vi "GA_Insert Into Population.vi"(6 "Parameters":T3={"Population size"=100, "Generations no."=500, "Significant digits"=4, "Crossover probabality"=0.85, "Mutation mode"=enum."one-point, fixed rate", "Use Gray code?"=FALSE, "Mutation rate"=0.05, "Min mutation rate"=0.0005, "Max mutation rate"=0.25, "Reproduction plan"=enum."Steady-state-replace-worst", "Elitism"=FALSE, "Fmax"=1} {"Max mutation rate" min=0.0 max=1.0; "Min mutation rate" min=0.0 max=1.0; "Mutation rate" min=0.0 max=1.0; "Crossover probabality" min=0.0 max=1.0; "Significant digits" min=1; "Generations no." min=1; "Population size" min=1}, 7 "Fitness Function":T2, 8 "Offsprings":i32[][](array[numeric]), 11 "Population in":T1) -> (3 "Population out":T1)   [LabVIEW 2016, in "Optimal Frequency Bands Search.lvlib" / "GeneticAlgorithm.lvlib"]
doc: "Вставить потомков в популяцию с учетом стратегии замещения особей (reproduction plan)"
uses:
  GeneticAlgorithm.lvlib
  GA_tParameters.ctl
  GA_tFitness Function.ctl
  GA_tPopulation.ctl
  particle_swarm_opt/ParticleSwarm.lvlib
panel:
  # "This VI is a part of BCI Design library, http://www.ru-bci.org \nCopyright © 2020, Sotnikov Peter, All rights reserved. License: CC BY-NC 4.0"
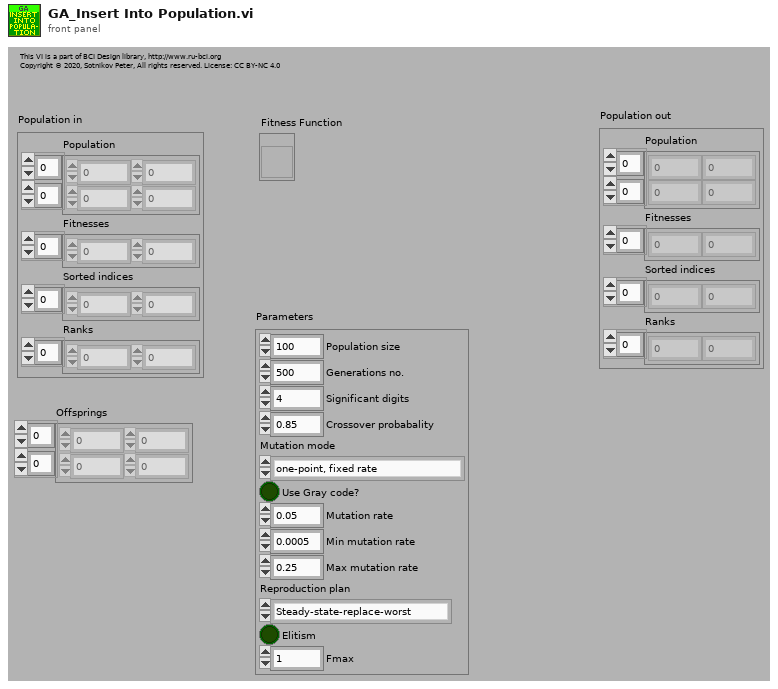
[diagram p1: front panel]
types:
  T1 = typedef "Optimal Frequency Bands Search.lvlib/GeneticAlgorithm.lvlib/GA_tPopulation.ctl" = cluster{"Population":i32[][], "Fitnesses":dbl[], "Sorted indices":i32[], "Ranks":i32[]}
  T2 = typedef "Optimal Frequency Bands Search.lvlib/GeneticAlgorithm.lvlib/GA_tFitness Function.ctl" = refnum<vi>
  T3 = typedef "Optimal Frequency Bands Search.lvlib/GeneticAlgorithm.lvlib/GA_tParameters.ctl" = cluster{"Population size":i32, "Generations no.":i32, "Significant digits":i32, "Crossover probabality":dbl, "Mutation mode":enum16{"one-point, fixed rate", "one-point, fitness-adjustable rate", "one-point, distance-adjustable rate"}, "Use Gray code?":bool, "Mutation rate":dbl, "Min mutation rate":dbl, "Max mutation rate":dbl, "Reproduction plan":enum16{"Full generational replacement", "Steady-state-replace-random", "Steady-state-replace-worst"}, "Elitism":bool, "Fmax":i32}
  T4 = enum16{"Full generational replacement", "Steady-state-replace-random", "Steady-state-replace-worst"}
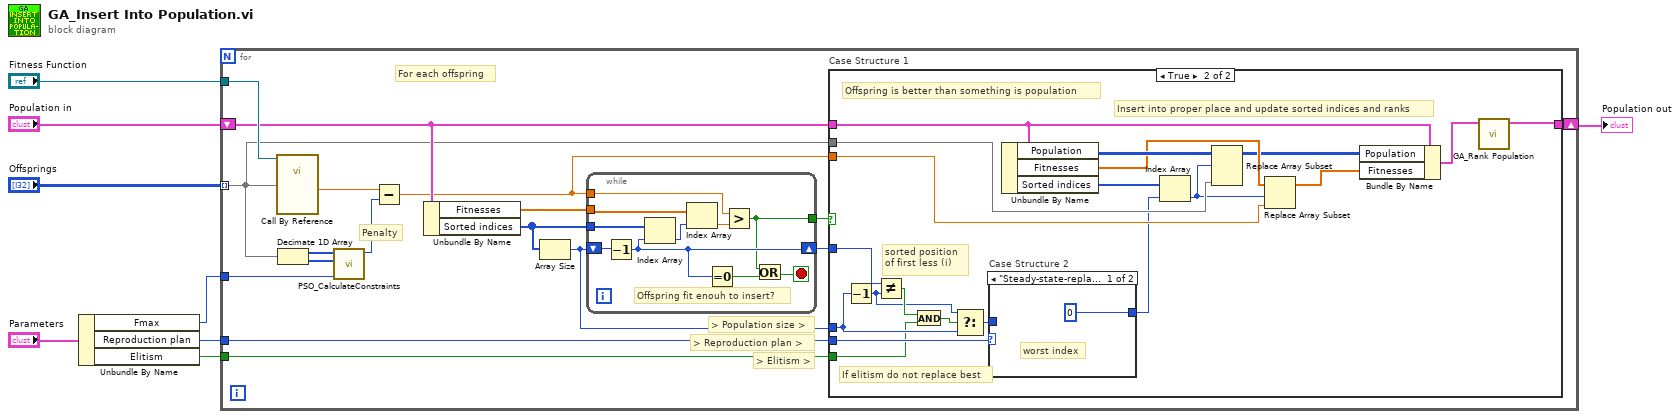
[diagram p0: block diagram]
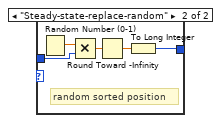
[diagram p3: hidden frame]
diagram:
  n1 = Unbundle By Name("Parameters") -> ("Fmax"=w1:i32, "Reproduction plan"=w5:T4, "Elitism"=w3:bool)
  n2 = for {
    tunnel: "Offsprings" -> [w14] mode=indexing
    shift-right: [w16] -> w2
    shift-left: "Population in" -> [w21]
    tunnel: w5 -> [w20]
    tunnel: "Fitness Function" -> [w25]
    tunnel: w3 -> [w18]
    tunnel: w1 -> [w15]
    # "Penalty"
    # "> Population size >"
    # "> Elitism >"
    # "> Reproduction plan >"
    # "For each offspring"
    n3 = call-by-ref "?"(reference=w25, "Phenotype"=w14) -> ("Fitness"=w9:dbl)  [unwired: 3 in, 2 out]
    n4 = Decimate 1D Array(w14) -> (w13:i32[], w12:i32[])
    n5 = call "PSO_CalculateConstraints.vi"("Fmax"=w15, "deltaF vector"=w12, "F0 vector"=w13) -> ("Penalty"=w11:i32)  [unwired: 7 in, 1 out]
    n6 = Subtract(x=w9, y=w11) -> (x-y=w10:dbl)
    n7 = Unbundle By Name(w21) -> ("Fitnesses"=w24:dbl[], "Sorted indices"=w23:i32[])
    n8 = Array Size(array=w23) -> (size(s)=w19:i32)
    n9 = while {
      tunnel: w24 -> [w60]
      tunnel: w23 -> [w61]
      shift-right: [w59] -> w17
      shift-left: w19 -> [w62]
      tunnel: w10 -> [w57]
      tunnel: [w54] -> w22
      stop <- w55 stop-if-true
      # "Offspring fit enouh to insert?"
      n10 = Decrement(x=w62) -> (x-1=w59:i32)
      n11 = Index Array(array=w61, index=w59) -> (element=w53:i32)
      n12 = Index Array(array=w60, index=w53) -> (element=w58:dbl)
      n13 = Equal To 0?(x=w59) -> (x = 0?=w56:bool)
      n14 = Greater?(x=w57, y=w58) -> (0:w54:bool)
      n15 = Or(x=w54, y=w56) -> (x .or. y?=w55:bool)
    }
    n16 = case "Case Structure 1" shown="True" w22 {
      tunnel: w21 -> [w26 w36]
      tunnel: w10 -> [_ w42]
      tunnel: w14 -> [_ w44]
      tunnel: w20 -> [_ w46]
      tunnel: w19 -> [_ w38]
      tunnel: w17 -> [_ w32]
      tunnel: w18 -> [_ w29]
      tunnel: [w26 w30] -> w16
      frame False {
        # "Offspring is worse than whole population"
      }
      frame True {
        # "Offspring is better than something is population"
        # "If elitism do not replace best"
        # "Insert into proper place and update sorted indices and ranks"
        # "sorted position \nof first less (i)"
        n17 = Decrement(x=w38) -> (x-1=w27:i32)
        n18 = Not Equal?(x=w32, y=w27) -> (x != y?=w40:bool)
        n19 = And(x=w40, y=w29) -> (x .and. y?=w39:bool)
        n20 = Select(t=w27, s=w39, f=w38) -> (s? t:f=w37:i32)
        n21 = case "Case Structure 2" shown="\"Steady-state-replace-worst\", Default" w46 {
          tunnel: w37 -> [_ w51]
          tunnel: [0 w48] -> w28
          frame "Steady-state-replace-worst", Default {
            # "worst index"
          }
          frame "Steady-state-replace-random" {
            # "random sorted position"
            n22 = Random Number (0-1)() -> (number: 0 to 1=w52:dbl)
            n23 = Multiply(x=w52, y=w51) -> (x*y=w50:dbl)
            n24 = Round Toward -Infinity(1:w50) -> (0:w49:dbl)
            n25 = To Long Integer(number=w49) -> (32bit integer=w48:i32)
          }
        }
        n26 = Unbundle By Name(w36) -> ("Population"=w45:i32[][], "Fitnesses"=w43:dbl[], "Sorted indices"=w41:i32[])
        n27 = Index Array(array=w41, index=w28) -> (element=w33:i32)
        n28 = Replace Array Subset(array=w45, new element=w44, index (row)=w33) -> (w35:i32[][])  [unwired: 1 in]
        n29 = Replace Array Subset(array=w43, new element=w42, index=w33) -> (w34:dbl[])
        n30 = Bundle By Name(cluster=w36, "Population"=w35, "Fitnesses"=w34) -> (w31:T1)
        n31 = call "GA_Rank Population.vi"("Population in"=w31) -> ("Population out"=w30:T1)  [unwired: 10 in]
      }
    }
  }
  "Population out" <- w2
